vi "format_status_response.vi"(10 "Response":string) -> (2 "Status cluster":T1)   [LabVIEW 2018]
uses:
  status_cluster.ctl
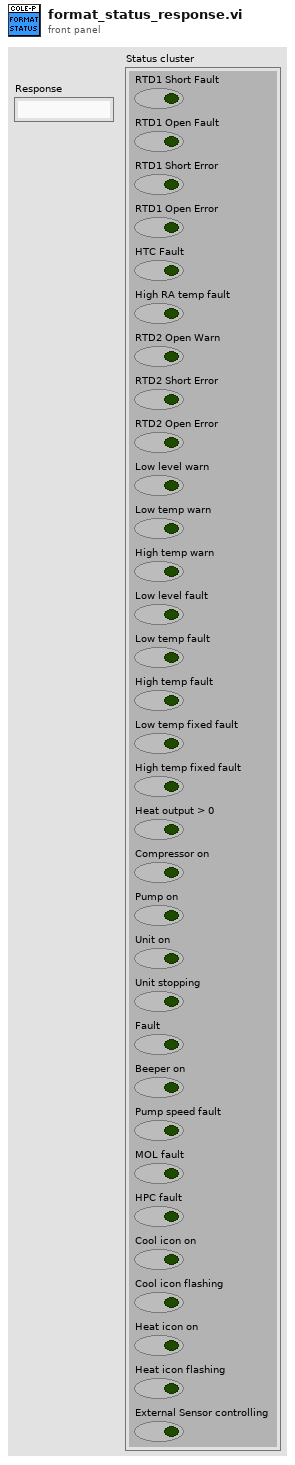
[diagram p1: front panel]
types:
  T1 = typedef "status_cluster.ctl" = cluster{"RTD1 Short Fault":bool, "RTD1 Open Fault":bool, "RTD1 Short Error":bool, "RTD1 Open Error":bool, "HTC Fault":bool, "High RA temp fault":bool, "RTD2 Open Warn":bool, "RTD2 Short Error":bool, "RTD2 Open Error":bool, "Low level warn":bool, "Low temp warn":bool, "High temp warn":bool, "Low level fault":bool, "Low temp fault":bool, "High temp fault":bool, "Low temp fixed fault":bool, "High temp fixed fault":bool, "Heat output > 0":bool, "Compressor on":bool, "Pump on":bool, "Unit on":bool, "Unit stopping":bool, "Fault":bool, "Beeper on":bool, "Pump speed fault":bool, "MOL fault":bool, "HPC fault":bool, "Cool icon on":bool, "Cool icon flashing":bool, "Heat icon on":bool, "Heat icon flashing":bool, "External Sensor controlling":bool}
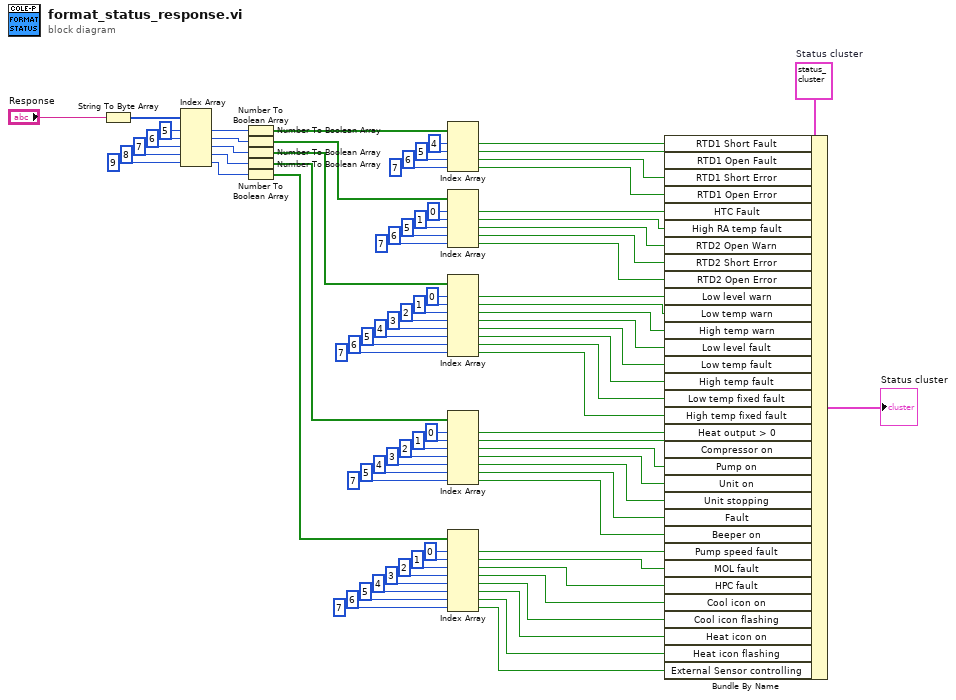
[diagram p0: block diagram]
diagram:
  w37 = T1 {"RTD1 Short Fault"=FALSE, "RTD1 Open Fault"=FALSE, "RTD1 Short Error"=FALSE, "RTD1 Open Error"=FALSE, "HTC Fault"=FALSE, "High RA temp fault"=FALSE, "RTD2 Open Warn"=FALSE, "RTD2 Short Error"=FALSE, "RTD2 Open Error"=FALSE, "Low level warn"=FALSE, "Low temp warn"=FALSE, "High temp warn"=FALSE, "Low level fault"=FALSE, "Low temp fault"=FALSE, "High temp fault"=FALSE, "Low temp fixed fault"=FALSE, "High temp fixed fault"=FALSE, "Heat output > 0"=FALSE, "Compressor on"=FALSE, "Pump on"=FALSE, "Unit on"=FALSE, "Unit stopping"=FALSE, "Fault"=FALSE, "Beeper on"=FALSE, "Pump speed fault"=FALSE, "MOL fault"=FALSE, "HPC fault"=FALSE, "Cool icon on"=FALSE, "Cool icon flashing"=FALSE, "Heat icon on"=FALSE, "Heat icon flashing"=FALSE, "External Sensor controlling"=FALSE}  # Status cluster
  n1 = String To Byte Array(string="Response") -> (unsigned byte array=w73:u8[])
  n2 = Index Array(array=w73, index #1=5 ("index"), index #2=6 ("index"), index #3=7 ("index"), index #4=8 ("index"), index #5=9 ("index")) -> (element #1=w79:u8, element #2=w80:u8, element #3=w81:u8, element #4=w82:u8, element #5=w83:u8)
  n3 = Number To Boolean Array(number=w79) -> (Boolean array=w71:bool[])
  n4 = Number To Boolean Array(number=w80) -> (Boolean array=w70:bool[])
  n5 = Number To Boolean Array(number=w81) -> (Boolean array=w69:bool[])
  n6 = Number To Boolean Array(number=w82) -> (Boolean array=w68:bool[])
  n7 = Number To Boolean Array(number=w83) -> (Boolean array=w38:bool[])
  n8 = Index Array(array=w71, index #1=4 ("index"), index #2=5 ("index"), index #3=6 ("index"), index #4=7 ("index")) -> (element #1=w36:bool, element #2=w32:bool, element #3=w31:bool, element #4=w30:bool)
  n9 = Index Array(array=w70, index #1=0 ("index"), index #2=1 ("index"), index #3=5 ("index"), index #4=6 ("index"), index #5=7 ("index")) -> (element #1=w29:bool, element #2=w28:bool, element #3=w27:bool, element #4=w26:bool, element #5=w25:bool)
  n10 = Index Array(array=w69, index #1=0 ("index"), index #2=1 ("index"), index #3=2 ("index"), index #4=3 ("index"), index #5=4 ("index"), index #6=5 ("index"), index #7=6 ("index"), index #8=7 ("index")) -> (element #1=w24:bool, element #2=w23:bool, element #3=w22:bool, element #4=w21:bool, element #5=w20:bool, element #6=w19:bool, element #7=w18:bool, element #8=w17:bool)
  n11 = Index Array(array=w68, index #1=0 ("index"), index #2=1 ("index"), index #3=2 ("index"), index #4=3 ("index"), index #5=4 ("index"), index #6=5 ("index"), index #7=7 ("index")) -> (element #1=w16:bool, element #2=w15:bool, element #3=w14:bool, element #4=w13:bool, element #5=w12:bool, element #6=w11:bool, element #7=w10:bool)
  n12 = Index Array(array=w38, index #1=0 ("index"), index #2=1 ("index"), index #3=2 ("index"), index #4=3 ("index"), index #5=4 ("index"), index #6=5 ("index"), index #7=6 ("index"), index #8=7 ("index")) -> (element #1=w9:bool, element #2=w8:bool, element #3=w7:bool, element #4=w6:bool, element #5=w5:bool, element #6=w4:bool, element #7=w3:bool, element #8=w2:bool)
  n13 = Bundle By Name(cluster=w37, "RTD1 Short Fault"=w36, "RTD1 Open Fault"=w32, "RTD1 Short Error"=w31, "RTD1 Open Error"=w30, "HTC Fault"=w29, "High RA temp fault"=w28, "RTD2 Open Warn"=w27, "RTD2 Short Error"=w26, "RTD2 Open Error"=w25, "Low level warn"=w24, "Low temp warn"=w23, "High temp warn"=w22, "Low level fault"=w21, "Low temp fault"=w20, "High temp fault"=w19, "Low temp fixed fault"=w18, "High temp fixed fault"=w17, "Heat output > 0"=w16, "Compressor on"=w15, "Pump on"=w14, "Unit on"=w13, "Unit stopping"=w12, "Fault"=w11, "Beeper on"=w10, "Pump speed fault"=w9, "MOL fault"=w8, "HPC fault"=w7, "Cool icon on"=w6, "Cool icon flashing"=w5, "Heat icon on"=w4, "Heat icon flashing"=w3, "External Sensor controlling"=w2) -> (→"Status cluster":T1)
